vi "WLAN_Descrambler.vi"(0 "scrambler initial bits":i8[](array[numeric]), 1 "data bits":i8[](array[numeric])) -> (6 "scrambled bits":i8[](array[numeric]))   [LabVIEW 2022 SP3]
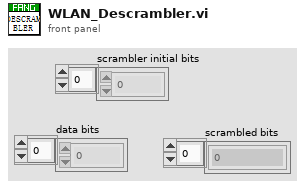
[diagram p1: front panel]
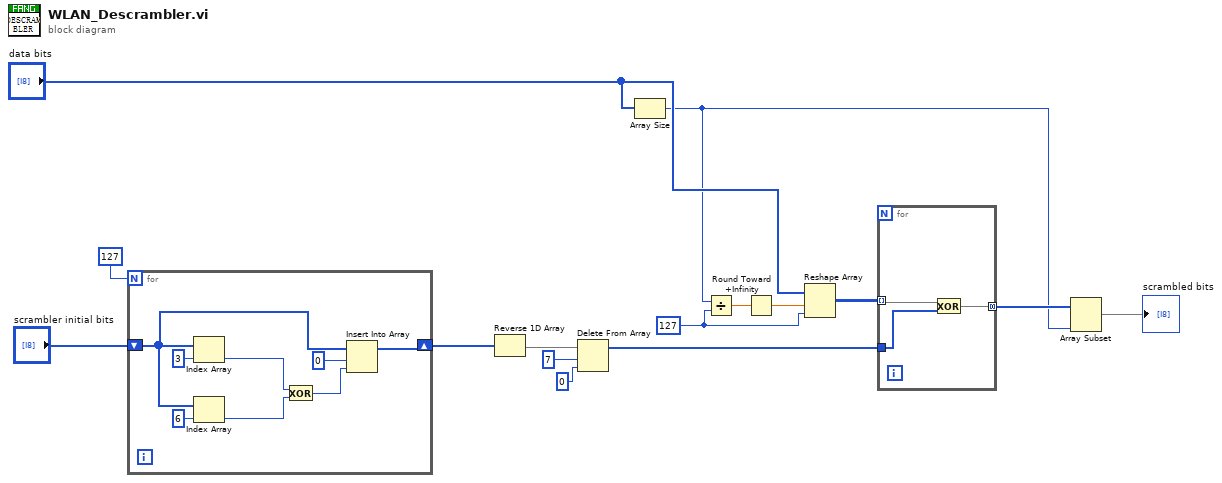
[diagram p0: block diagram]
diagram:
  w2 = 127
  n1 = for {
    N: 127 -> [_]
    shift-right: [w16] -> w5
    shift-left: "scrambler initial bits" -> [w19]
    n2 = Index Array(array=w19, index=3) -> (element=w21:i8)
    n3 = Index Array(array=w19, index=6) -> (element=w20:i8)
    n4 = Exclusive Or(1:w20, 2:w21) -> (0:w17:i8)
    n5 = Insert Into Array(array=w19, index=0, new element=w17) -> (w16:i8[])
  }
  n6 = Reverse 1D Array(array=w5) -> (reversed array=w6:i8[])
  n7 = Delete From Array(array=w6, length=7, index=0) -> (array with subset deleted=w15:i8[])  [unwired: 1 out]
  n8 = Array Size(array="data bits") -> (size(s)=w10:i32)
  n9 = Divide(x=w10, y=w2) -> (x/y=w4:dbl)
  n10 = Round Toward +Infinity(x=w4) -> (ceil(x): smallest int >= x=w3:dbl)
  n11 = Reshape Array("data bits", w3, w2) -> (w1:i8[][])
  n12 = for {
    tunnel: w1 -> [w24] mode=indexing
    tunnel: w15 -> [w26]
    tunnel: [w25] -> w12 mode=concatenating
    n13 = Exclusive Or(1:w26, 2:w24) -> (0:w25:i8[])
  }
  n14 = Array Subset(array=w12, length=w10) -> (→"scrambled bits":i8[])  [unwired: 1 in]
